vi "Logging Stopped.vi"(8 "error in (no error)":errorcluster, 10 "Context in":refnum<class "Context.lvclass">, 11 "Logging in":refnum<class "Logging.lvclass">) -> (0 "error out":errorcluster, 2 "Context out":refnum<class "Context.lvclass">, 3 "State out":refnum<class "State.lvclass">)   [LabVIEW 2024, in "State.lvlib" / "Logging.lvclass"]
uses:
  Logging.lvclass
  C:/Users/uspoaotto/OneDrive - Oregon Tool/Desktop/working copies/stateMachineActor/src/State Machine/State/State/State.lvclass
  Context/Context/Context.lvclass
  State/State.lvclass
  Logging.lvclass/Logging.ctl
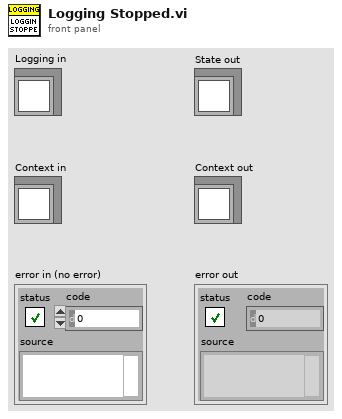
[diagram p1: front panel]
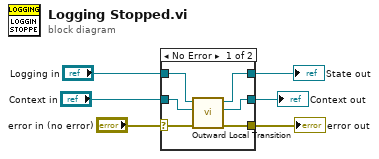
[diagram p0: block diagram]
diagram:
  n1 = case shown="No Error" "error in (no error)" {
    selector: "error in (no error)" -> [w7 w15]
    tunnel: "Logging in" -> [w12 w13]
    tunnel: "Context in" -> [w11 w14]
    tunnel: [w10 w13] -> w1
    tunnel: [w9 w14] -> w4
    tunnel: [w8 w15] -> w3
    frame No Error {
      n2 = call "Outward Local Transition.vi"("error in (no error)"=w7, "Context in"=w11, "State in"=w12) -> ("error out"=w8:errorcluster, "Context out"=w9:refnum<class "Context.lvclass">, "State out"=w10:refnum<class "State.lvclass">)  [unwired: 6 in]
    }
    frame Error {
    }
  }
  "error out" <- w3
  "Context out" <- w4
  "State out" <- w1
